vi "FPGA SPI_FPGA Top Level.vi"() -> ()   [LabVIEW 2019]
uses:
  spi_example/FPGA/Controls/FPGA SPI_FPGA SPI State.ctl
  spi_example/FPGA/Controls/FPGA SPI_Communication Loop State.ctl
  <vilib>/rvi/Emulation/niFpgaGetClockAttributes.vi
  <vilib>/rvi/Emulation/niFpgaSctlEmulationGetInTimedLoop.vi
  <vilib>/rvi/Emulation/niFpgaEmulationReportErrorSimple.vi
  spi_example/FPGA/Code/FPGA SPI_Globals.vi
  <vilib>/rvi/Emulation/niFpgaProcessEmulError.vi
  <vilib>/rvi/Emulation/niFpgaCriticalErrorInLSC.vi
  <vilib>/rvi/Emulation/niFpgaEmulationIsFPGAContextNoSignature.vi
  <vilib>/rvi/errors/niFpgaSetErrorForExecOnDevCompSimple.vi
  <vilib>/rvi/eio/common/nirviEmuReportErrorAndStop.vi
  <vilib>/rvi/DataTransferAndStorage/Container/Common/niFpgaContainerGetUniqueNameForEmu.vi
  <vilib>/rvi/FIFO/Fifo_Resource/nirvififoEmulationSetSize.vi
  <vilib>/rvi/FIFO/Fifo_Resource/nirviFifoEmulationQueueMgr.vi
  <instcachedir>/0/nirviFifoEmulationQueueMgr_E5CAEC123FF24DC58D834DCA3CDAA9B5.lvgen/nirviFifoEmulationQueueMgr_E5CAEC123FF24DC58D834DCA3CDAA9B5_002.vi
  <vilib>/rvi/FIFO/Fifo_Resource/nirvififoEmulationDetermineInputValidOut.vi
  <vilib>/rvi/FIFO/Fifo_Resource/nirvififoEmulationCreateLock.vi
  <vilib>/rvi/FIFO/Fifo_Resource/nirvififoEmulationObtainLock.vi
  <vilib>/rvi/FIFO/Fifo_Resource/nirvififoEmulationReleaseLock.vi
  <vilib>/rvi/occurrence/nirviWaitOnOccurrenceBase.vi
  <vilib>/rvi/errors/nirviReportUnexpectedCaseInternalError.vi
  <vilib>/rvi/errors/nirviReportUnexpectedCaseInternalError (U32).vi
  <vilib>/Utility/error.llb/Clear Errors.vi
  <vilib>/rvi/DataTransferAndStorage/Container/XNode/niFpgaContainer.xnode
  <vilib>/rvi/FIFO/Fifo_Resource/nirvififoEmulationWrite.vi
  <vilib>/rvi/FIFO/Fifo_Resource/nirvififoEmulationRead.vi
panel:
  in  "SPI_Clock Divider":u32=20
  in  "SPI_CS Active State":bool caption="SPI_CS\nActive State"
  in  "SPI_CPOL":bool
  in  "SPI_CPHA":bool
  in  "SPI_CS":u8=1 format="%08b"
  in  "SPI_Total Bits":u16=8
  in  "SPI_Total Bytes":u16=1
  in  "SPI_Start":bool
  in  "SPI_Cmd":T1
  in  "SPI_Ack Read":bool
  out "SPI_Read Data":u8
  out "SPI_Read Flag":bool
  in  "SPI_Write Flag":bool
  in  "SPI_Write Data":u8
  in  "SPI_Port":i8
  # "Control"
  # "SPI Configuration Parameters"
  # "Command Type"
  # "Host Data Transfer"
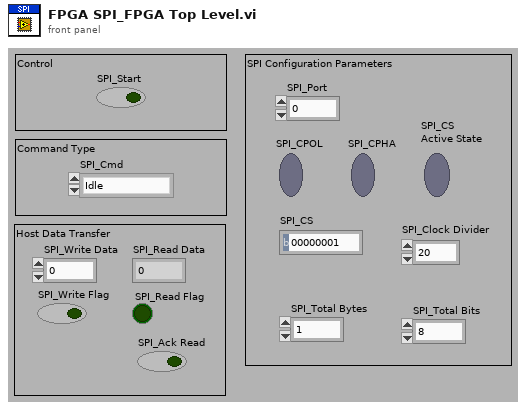
[diagram p1: front panel]
types:
  T1 = typedef "FPGA SPI_FPGA SPI State.ctl" = enum8{"Idle", "Read/Write SPI", "Configure"}
  T2 = cluster{"SCLK":refnum<k21>, "CS":refnum<k21>, "MOSI":refnum<k21>, "MISO":refnum<k21>}
  T3 = typedef "FPGA SPI_Communication Loop State.ctl" = enum8{"Idle", "Init", "Write", "Start", "Read", "Wait Until Done"}
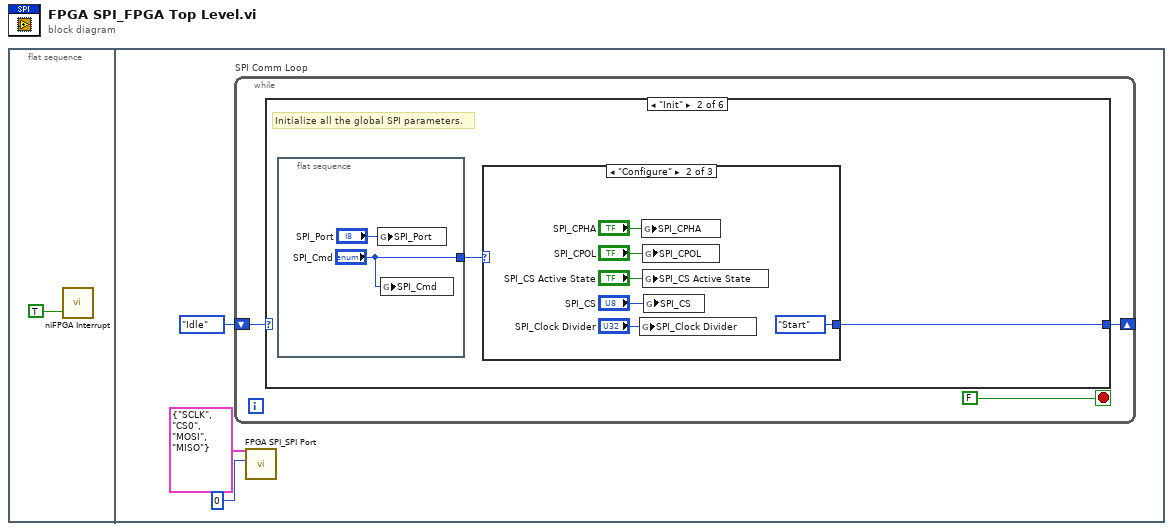
[diagram p0: block diagram]
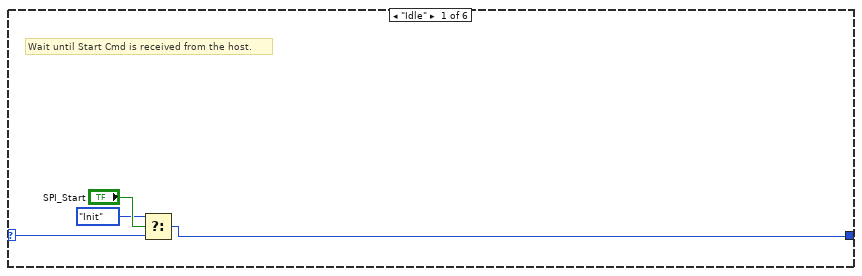
[diagram p2: hidden frame]
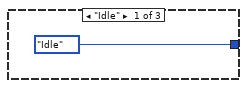
[diagram p3: hidden frame]
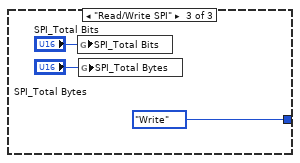
[diagram p4: hidden frame]
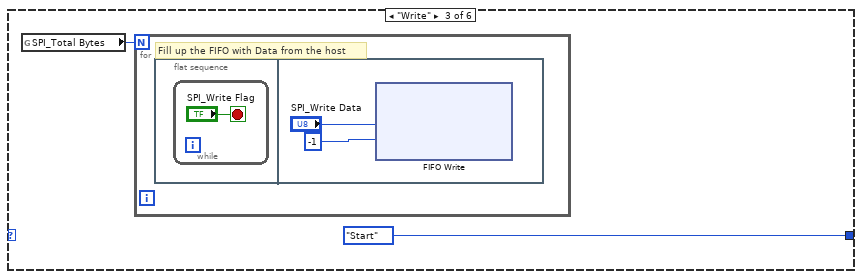
[diagram p5: hidden frame]
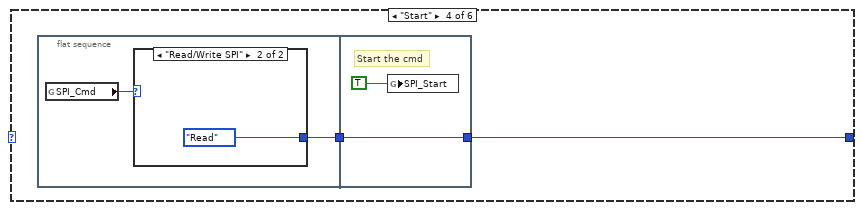
[diagram p6: hidden frame]
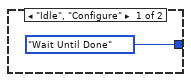
[diagram p7: hidden frame]
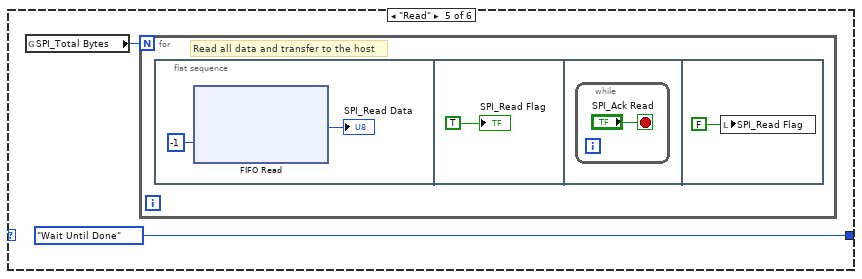
[diagram p8: hidden frame]
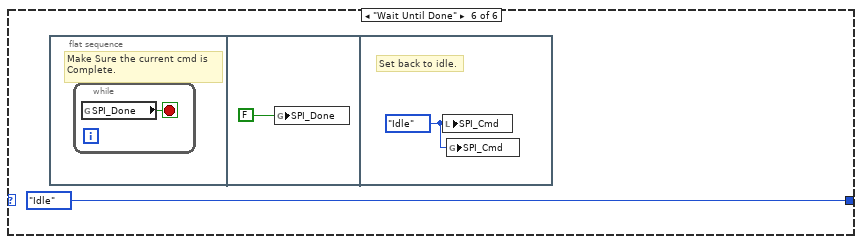
[diagram p9: hidden frame]
diagram:
  n1 = flat-sequence {
    frame #0 {
      n2 = call <vilib>:"niFPGA Interrupt.vi"("Wait Until Cleared (F)"=TRUE ("Wait Until Cleared")) -> ()  [unwired: 2 in]
    }
    frame #1 {
      n3 = while "SPI Comm Loop" {
        shift-right: [w6] -> _
        shift-left: FPGA_SPI_Communication_Loop_State."Idle" ("Action") -> [w5]
        stop <- FALSE stop-if-true
        n4 = case shown="\"Init\"" w5 {
          selector: w5 -> [w10 _ _ _ _ _]
          tunnel: [w8 w12 FPGA_SPI_Communication_Loop_State."Start" ("Action") w32 FPGA_SPI_Communication_Loop_State."Wait Until Done" ("Action") FPGA_SPI_Communication_Loop_State."Idle" ("Action")] -> w6
          frame "Idle" {
            # "Wait until Start Cmd is received from the host."
            n5 = Select(t=FPGA_SPI_Communication_Loop_State."Init" ("Action"), s="SPI_Start", f=w10) -> (s? t:f=w8:T3)
          }
          frame "Init" {
            # "Initialize all the global SPI parameters."
            n6 = flat-sequence {
              tunnel: ["SPI_Cmd"] -> w13
              frame #0 {
                n7 = global write "FPGA SPI_Globals.vi" "SPI_Port"("SPI_Port") -> ()
                n8 = global write "FPGA SPI_Globals.vi" "SPI_Cmd"("SPI_Cmd") -> ()
              }
            }
            n9 = case shown="\"Configure\"" w13 {
              tunnel: [FPGA_SPI_Communication_Loop_State."Idle" ("Action") FPGA_SPI_Communication_Loop_State."Start" ("Action") FPGA_SPI_Communication_Loop_State."Write" ("Action")] -> w12
              frame "Idle" {
              }
              frame "Configure" {
                n10 = global write "FPGA SPI_Globals.vi" "SPI_Clock Divider"("SPI_Clock Divider") -> ()
                n11 = global write "FPGA SPI_Globals.vi" "SPI_CPHA"("SPI_CPHA") -> ()
                n12 = global write "FPGA SPI_Globals.vi" "SPI_CPOL"("SPI_CPOL") -> ()
                n13 = global write "FPGA SPI_Globals.vi" "SPI_CS Active State"("SPI_CS Active State") -> ()
                n14 = global write "FPGA SPI_Globals.vi" "SPI_CS"("SPI_CS") -> ()
              }
              frame "Read/Write SPI" {
                n15 = global write "FPGA SPI_Globals.vi" "SPI_Total Bits"("SPI_Total Bits") -> ()
                n16 = global write "FPGA SPI_Globals.vi" "SPI_Total Bytes"("SPI_Total Bytes") -> ()
              }
            }
          }
          frame "Write" {
            n17 = global read "FPGA SPI_Globals.vi" "SPI_Total Bytes"() -> (w27:u16)
            n18 = for {
              N: w27 -> [_]
              # "Fill up the FIFO with Data from the host"
              n19 = flat-sequence {
                frame #0 {
                  n20 = while {
                    stop <- "SPI_Write Flag" stop-if-true
                  }
                }
                frame #1 {
                  n21 = xnode ("FIFO Write")("Element"="SPI_Write Data", "Timeout"=-1) -> ()  [unwired: 1 in, 2 out]
                }
              }
            }
          }
          frame "Start" {
            n22 = flat-sequence {
              tunnel: [w33] -> w31
              tunnel: [w38] -> w32
              tunnel: w31 -> [w38]
              frame #0 {
                n23 = global read "FPGA SPI_Globals.vi" "SPI_Cmd"() -> (w34:T1)
                n24 = case shown="\"Read/Write SPI\"" w34 {
                  tunnel: [FPGA_SPI_Communication_Loop_State."Wait Until Done" ("Action") FPGA_SPI_Communication_Loop_State."Read" ("Action")] -> w33
                  frame "Idle", "Configure" {
                  }
                  frame "Read/Write SPI" {
                  }
                }
              }
              frame #1 {
                # "Start the cmd"
                n25 = global write "FPGA SPI_Globals.vi" "SPI_Start"(TRUE ("Write Flag")) -> ()
              }
            }
          }
          frame "Read" {
            n26 = global read "FPGA SPI_Globals.vi" "SPI_Total Bytes"() -> (w40:u16)
            n27 = for {
              N: w40 -> [_]
              # "Read all data and transfer to the host"
              n28 = flat-sequence {
                frame #0 {
                  n29 = xnode ("FIFO Read")("Timeout"=-1) -> ("Element"=→"SPI_Read Data":u8)  [unwired: 1 in, 2 out]
                }
                frame #1 {
                  "SPI_Read Flag" <- TRUE ("Read Flag")
                }
                frame #2 {
                  n30 = while {
                    stop <- "SPI_Ack Read" stop-if-true
                  }
                }
                frame #3 {
                  n31 = local write "SPI_Read Flag"(FALSE ("Read Flag")) -> ()
                }
              }
            }
          }
          frame "Wait Until Done" {
            n32 = flat-sequence {
              frame #0 {
                # "Make Sure the current cmd is\nComplete."
                n33 = while {
                  stop <- w47 stop-if-true
                  n34 = global read "FPGA SPI_Globals.vi" "SPI_Done"() -> (w47:bool)
                }
              }
              frame #1 {
                n35 = global write "FPGA SPI_Globals.vi" "SPI_Done"(FALSE ("Done")) -> ()
              }
              frame #2 {
                w49 = FPGA_SPI_FPGA_SPI_State."Idle" ("Type")
                # "Set back to idle."
                n36 = local write "SPI_Cmd"(w49) -> ()
                n37 = global write "FPGA SPI_Globals.vi" "SPI_Cmd"(w49) -> ()
              }
            }
          }
        }
      }
      n38 = call "FPGA SPI_SPI Port.vi"("Port"=i8 0, "FPGA IO"=T2 {"SCLK"="SCLK", "CS"="CS0", "MOSI"="MOSI", "MISO"="MISO"}) -> ()  [unwired: 10 out]
    }
  }
